vi "fmTest_MQTT_Simple_Connect_and_Subscribe.vi"() -> ()   [LabVIEW 2018]
doc: "A basic client example that connects to a server, subscribes to a variety of topics and receives responses for the topics. \n\n© 2015 - daq.io, LLC - Peter Adelhardt"
uses:
  source/support/mqtt/Controls/Connect_Flags.ctl
  source/support/mqtt/Controls/QoS.ctl
  source/support/mqtt/Controls/Connection_Return_Codes.ctl
  source/support/mqtt/Controls/MessageType.ctl
  source/support/mqtt/Controls/DUP_Flag.ctl
  source/support/mqtt/Controls/Retain_Flag.ctl
  source/support/mqtt/MQTT_Functions.lvlib
panel:
  in  "Message ID":u16=10
  in  "timeout ms (25000)":i32=1000
  out "timeout count":i32
  out "mSec":u32
  out "message count":i32
  out "Last message":T2
  in  "Stop Reading":bool
  in  "MQTT Broker":cluster{"address (IP)":string, "port":u16}={"address (IP)"="10.96.1.58", "port"=1883}
  in  "Subscription Info Array":cluster{"Topic":string, "QoS":T3}[](array[cluster])=[{"Topic"="a/b", "QoS"=enum."At most once"}]
  out "Granted QoS Levels":T3[](array[typedef])
  out "Connection Status":T4=enum."Connection refused: Server unavailable"
  in  "Connect Flags":T5
  in  "Client ID":string="LVSubscribeClient2"
  out "error out":errorcluster
  in  "error in (no error)":errorcluster
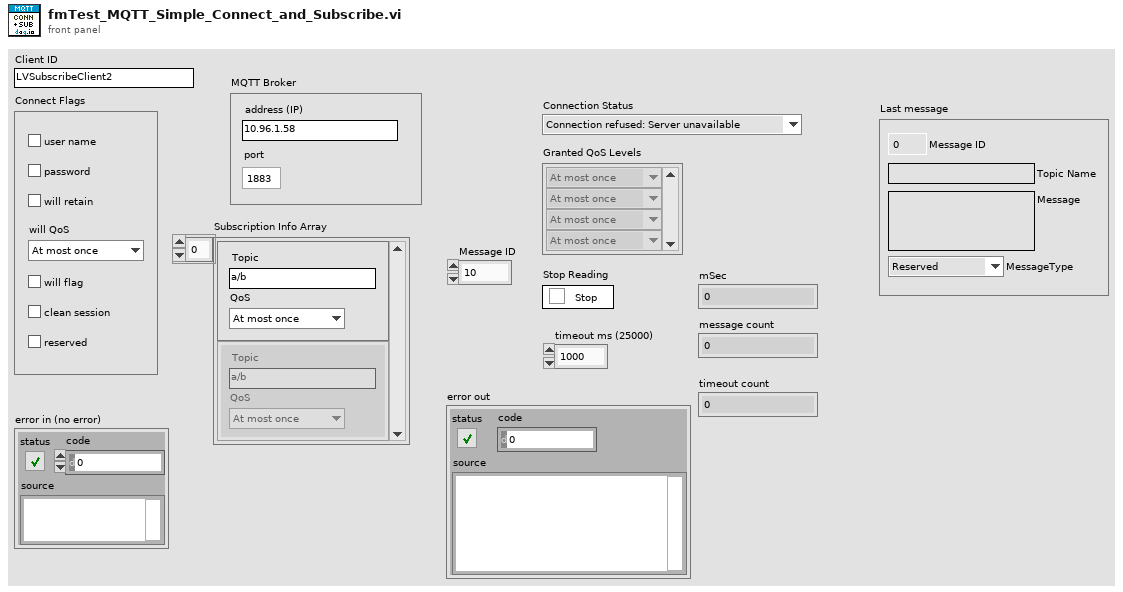
[diagram p1: front panel]
types:
  T1 = typedef "MQTT_Functions.lvlib/MessageType.ctl" = enum32{"Reserved", "CONNECT", "CONNACK", "PUBLISH", "PUBACK", "PUBREC", "PUBREL", "PUBCOMP", "SUBSCRIBE", "SUBACK", "UNSUBSCRIBE", "UNSUBACK", "PINGREQ", "PINGRESP", "DISCONNECT", "Reserved2"}
  T2 = cluster{"Message ID":u16, "Topic Name":string, "Message ":string, "MessageType":T1}
  T3 = typedef "MQTT_Functions.lvlib/QoS.ctl" = enum8{"At most once", "At least once", "Exactly once", "Reserved"}
  T4 = typedef "MQTT_Functions.lvlib/Connection_Return_Codes.ctl" = enum16{"Connection accepted", "Connection refused: unacceptable protocol version", "Connection refused: identifier rejected", "Connection refused: Server unavailable", "Connection refused: bad user name or password", "Connection refused: not authorized"}
  T5 = typedef "MQTT_Functions.lvlib/Connect_Flags.ctl" = cluster{"user name":bool, "password":bool, "will retain":bool, "will flag":bool, "clean session":bool, "reserved":bool, "will QoS":T3}
  T6 = typedef "MQTT_Functions.lvlib/DUP_Flag.ctl" = bool
  T7 = typedef "MQTT_Functions.lvlib/Retain_Flag.ctl" = bool
  T8 = cluster{"QoS":T3, "DUP":T6, "Retain":T7, "Keep Alive (sec)":u16}
  T9 = cluster{"Message ID":u16, "Topic Name":string, "Message":string, "MessageType":T1}
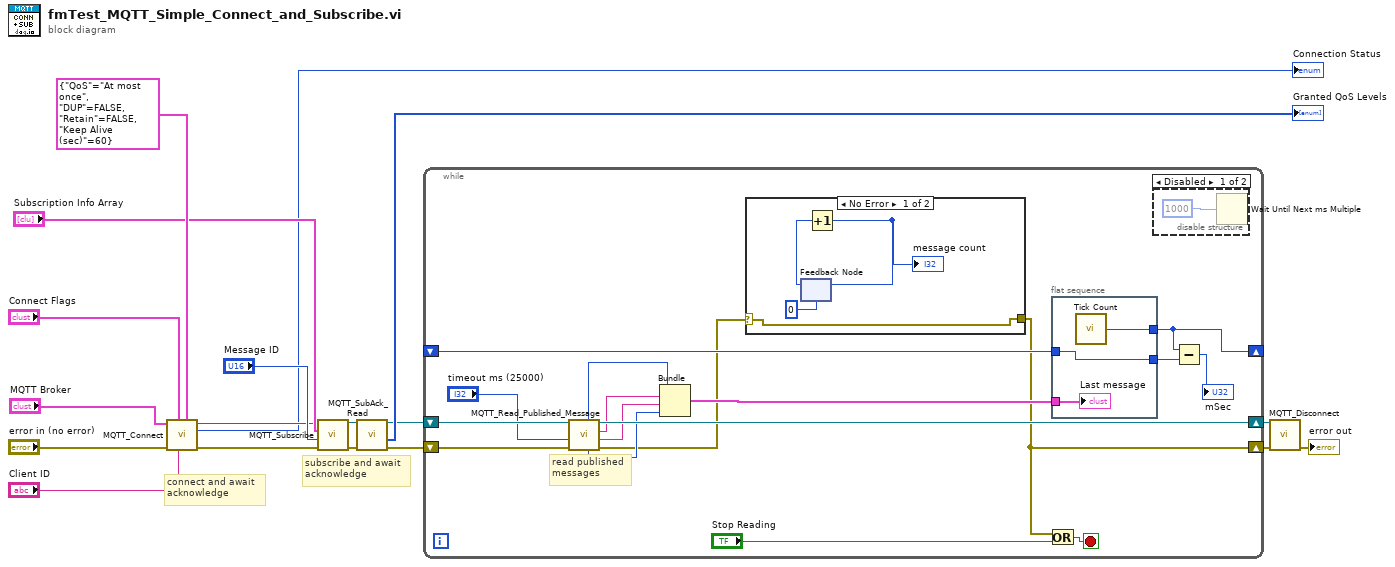
[diagram p0: block diagram]
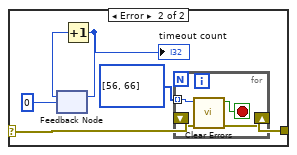
[diagram p2: hidden frame]
diagram:
  # "connect and await\nacknowledge"
  # "subscribe and await\nacknowledge"
  n1 = call "MQTT_Connect.vi"("Connect Meta"=T8 {"QoS"=enum."At most once", "DUP"=FALSE, "Retain"=FALSE, "Keep Alive (sec)"=60}, "Client ID"="Client ID", "Connect Flags"="Connect Flags", "error in (no error)"="error in (no error)", "MQTT Broker"="MQTT Broker") -> ("error out"=w1:errorcluster, "Connection Status"=→"Connection Status":T4, "connection ID out"=w3:refnum<k5>)  [unwired: 4 in]
  n2 = call "MQTT_Subscribe.vi"("error in (no error)"=w1, "Message ID"="Message ID", "Subscription Info Array"="Subscription Info Array", "connection ID"=w3) -> ("error out"=w11:errorcluster, "connection ID out"=w12:refnum<k5>)  [unwired: 6 in]
  n3 = call "MQTT_SubAck_Read.vi"("error in (no error)"=w11, "connection ID"=w12) -> ("error out"=w9:errorcluster, "Granted QoS Levels"=→"Granted QoS Levels":T3[], "connection ID out"=w8:refnum<k5>)  [unwired: 7 in]
  n4 = while {
    shift-right: [w20] -> w6
    shift-left: w9 -> [w35]
    shift-right: [w33] -> w7
    shift-left: w8 -> [w34]
    shift-right: [w24] -> _
    shift-left: _ -> [w25]
    stop <- w28 stop-if-true
    # "read published\nmessages"
    n5 = call "MQTT_Read_Published_Message.vi"("error in (no error)"=w35, "timeout ms (25000)"="timeout ms (25000)", "connection ID"=w34) -> ("error out"=w21:errorcluster, "Message"=w30:string, "Topic Name"=w31:string, "connection ID out"=w33:refnum<k5>, "MessageType"=w29:T1, "Message ID"=w32:u16)  [unwired: 3 in]
    n6 = Bundle("Message ID"=w32, "Topic Name"=w31, "Message"=w30, "MessageType"=w29) -> (w26:T9)  [unwired: 1 in]
    n7 = case shown="No Error" w21 {
      selector: w21 -> [w36 w45]
      tunnel: [w36 w44] -> w20
      frame No Error {
        n8 = feedback #1(0) -> (w39:i32)
        n9 = Increment(x=w39) -> (x+1=w38:i32)
        "message count" <- w38
        n10 = feedback-in #1(w38) -> ()
      }
      frame Error {
        n11 = feedback #2(0) -> (w42:i32)
        n12 = Increment(x=w42) -> (x+1=w41:i32)
        "timeout count" <- w41
        n13 = feedback-in #2(w41) -> ()
        n14 = for {
          tunnel: i32[] [56, 66] ("specific error code to clear (0: all)") -> [w47] mode=indexing
          shift-right: [w48] -> w44
          shift-left: w45 -> [w49]
          stop <- w46 stop-if-true
          n15 = call <vilib>:"Clear Errors.vi"("error in (no error)"=w49, "specific error code to clear (0: all)"=w47) -> ("error out"=w48:errorcluster, "specific error cleared?"=w46:bool)  [unwired: 4 in]
        }
      }
    }
    n16 = Or(x=w20, y="Stop Reading") -> (x .or. y?=w28:bool)
    n17 = flat-sequence {
      tunnel: w26 -> [w52]
      tunnel: [w51] -> w24
      tunnel: w25 -> [w50]
      tunnel: [w50] -> w23
      frame #0 {
        n18 = call "Tick Count"() -> ("Tick Count(mSec)"=w51:u32)
        "Last message" <- w52
      }
    }
    n19 = disable-structure shown="Disabled" {
      frame Disabled {
        n20 = Wait Until Next ms Multiple(millisecond multiple=u32 1000) -> ()  [unwired: 1 out]
      }
      frame Enabled {
      }
    }
    n21 = Subtract(x=w24, y=w23) -> (x-y=→"mSec":u32)
  }
  n22 = call "MQTT_Disconnect.vi"("error in (no error)"=w6, "connection ID"=w7) -> ("error out"=→"error out":errorcluster)  [unwired: 9 in]
